vi "Log Result.vi"(8 "error in (no error)":errorcluster, 10 "tdms file":refnum<k34>, 11 "DBL Result in":refnum<class "DBL Result.lvclass">) -> (0 "error out":errorcluster, 2 "tdms file out":refnum<k34>, 3 "DBL Result out":refnum<class "DBL Result.lvclass">)   [LabVIEW 2015, in "DBL Result.lvclass"]
uses:
  DBL Result.lvclass
  Mag Lab Result.lvclass/Mag Lab Result.ctl
  Read Group Name.vi
  Read Name.vi
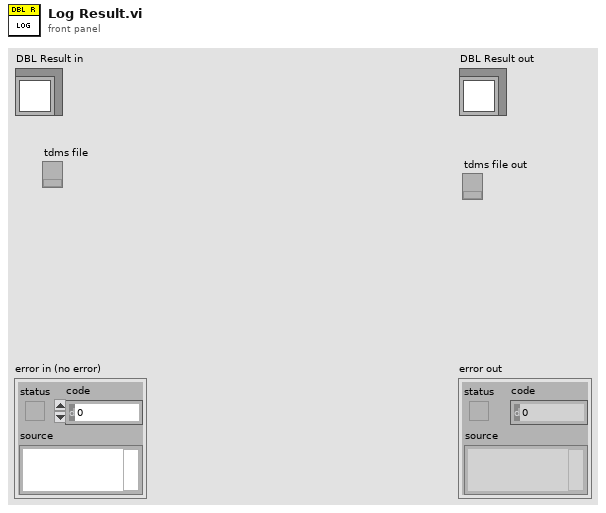
[diagram p1: front panel]
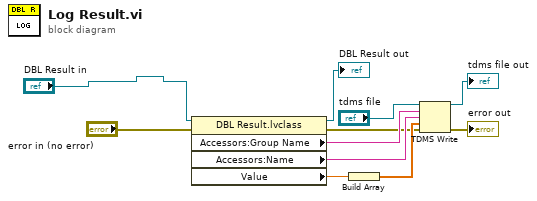
[diagram p0: block diagram]
diagram:
  n1 = property class="DBL Result.lvclass"(reference="DBL Result in", error in="error in (no error)") -> (reference out=→"DBL Result out":refnum<class "DBL Result.lvclass">, error out=w3:errorcluster, "Accessors:Group Name"=w6:string, "Accessors:Name"=w7:string, "Value"=w5:dbl)
  n2 = Build Array(w5) -> (w8:dbl[])
  n3 = TDMS Write(0:"tdms file", 5:w6, 7:w7, 9:w8, 11:w3) -> (4:→"tdms file out":refnum<k34>, 15:→"error out":errorcluster)  [unwired: 1 in, 2 out]
